vi "Logging Writing Cache.vi"(4 "error in (no error)":errorcluster, 5 "Variable":T2, 6 "Mode":T3, 7 "LoggingDevRef":T1) -> (0 "error out":errorcluster, 1 "Out":T2[](array[typedef]), 3 "LoggingDevRef":T1)   [LabVIEW 2012, in "femtoRoboLib.lvlib"]
uses:
  femtoRoboLib.lvlib
  Controls/Log Entry - Converted.ctl
  Controls/Logging Cache - Mode.ctl
  Controls/LoggingDevRef.ctl
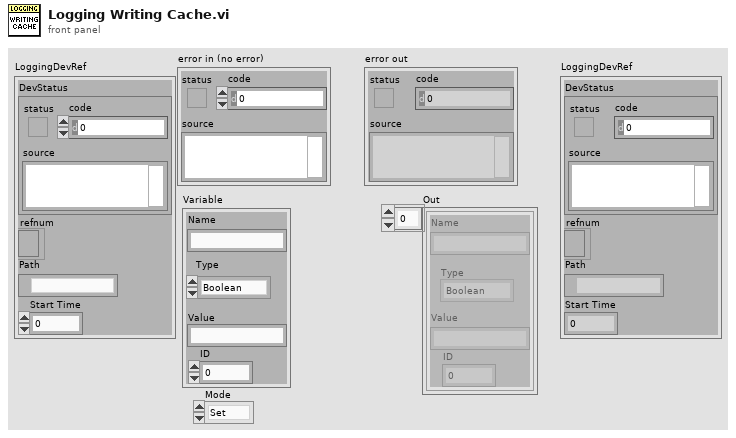
[diagram p1: front panel]
types:
  T1 = typedef "femtoRoboLib.lvlib/LoggingDevRef.ctl" = cluster{"DevStatus":errorcluster, "refnum":refnum<file>, "Path":path, "Start Time":u32}
  T2 = typedef "femtoRoboLib.lvlib/Log Entry - Converted.ctl" = cluster{"Name":string, "Type":enum16{"Boolean", "Numeric", "String", "Boolean Array", "Numeric Array", "String Array"}, "Value":string, "ID":u32}
  T3 = typedef "Logging Cache - Mode.ctl" = enum16{"Set", "Get All", "Get Unsaved", "Get Unsaved and Clear", "Get New", "Get New and Clear"}
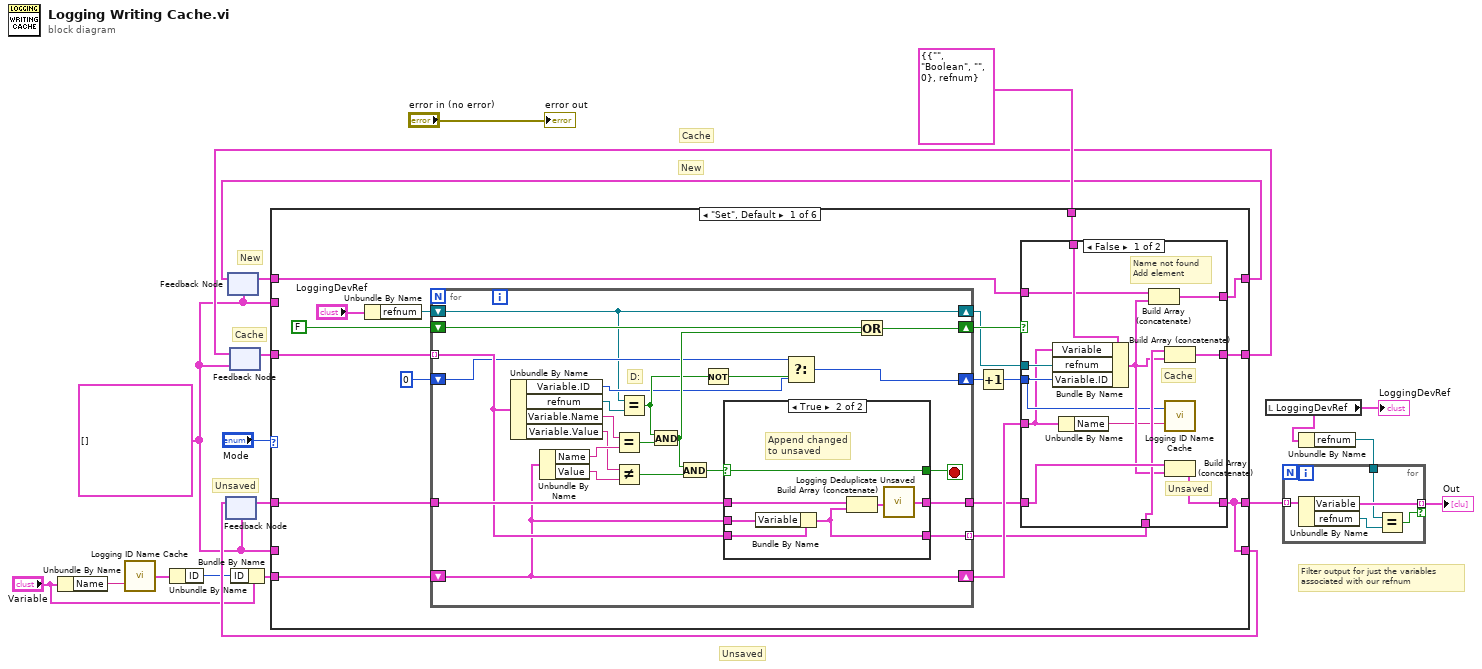
[diagram p0: block diagram]
diagram:
  w7 = cluster{"Variable":T2, "refnum":refnum<file>}[] [] ("Cache")
  # "New"
  # "Cache"
  # "Unsaved"
  # "New"
  # "Cache"
  # "Filter output for just the variables\nassociated with our refnum"
  # "Unsaved"
  n1 = Unbundle By Name("Variable") -> ("Name"=w5:string)
  n2 = call "Logging ID Name Cache.vi"("Name"=w5) -> ("ID/Name"=w4:cluster{"ID":u32, "Name":string})  [unwired: 1 in]
  n3 = Unbundle By Name(w4) -> ("ID"=w2:u32)
  n4 = feedback #1(w7) -> (w18:cluster{"Variable":T2, "refnum":refnum<file>}[])
  n5 = feedback #2(w7) -> (w8:cluster{"Variable":T2, "refnum":refnum<file>}[])
  n6 = feedback #3(w7) -> (w19:cluster{"Variable":T2, "refnum":refnum<file>}[])
  n7 = Bundle By Name(cluster="Variable", "ID"=w2) -> (w1:T2)
  n8 = case shown="\"Set\", Default" "Mode" {
    tunnel: w19 -> [w31 w88 w91 w94 w98 w102]
    tunnel: w18 -> [w38 w89 w92 w95 w99 w103]
    tunnel: [w33 w88 w92 w95 w97 w101] -> w13
    tunnel: w7 -> [_ _ _ w96 _ _]
    tunnel: [w33 w89 w92 w96 w99 w103] -> w16
    tunnel: cluster{"Variable":T2, "refnum":refnum<file>} {"Variable"={"Name"="", "Type"=enum."Boolean", "Value"="", "ID"=0}, "refnum"=refnum} ("Cache Entry") -> [w32 _ _ _ _ _]
    tunnel: [w30 w88 w91 w94 w98 w102] -> w14
    tunnel: w8 -> [w24 w87 w90 w93 w97 w101]
    tunnel: [w25 w87 w90 w93 w97 w100] -> w6
    tunnel: w7 -> [_ _ _ _ _ w100]
    tunnel: w1 -> [w23 _ _ _ _ _]
    frame "Set", Default {
      n9 = Unbundle By Name("LoggingDevRef") -> ("refnum"=w22:refnum<file>)
      n10 = for {
        tunnel: w31 -> [w63] mode=indexing
        tunnel: [w71] -> w34
        tunnel: w38 -> [w72]
        shift-right: [w69] -> w35
        shift-left: FALSE -> [w70]
        tunnel: [w62] -> w29 mode=indexing
        shift-right: [w59] -> w27
        shift-left: u32 0 -> [w56]
        shift-right: [w55] -> w36
        shift-left: w23 -> [w55]
        shift-right: [w54] -> w21
        shift-left: w22 -> [w54]
        stop <- w61 stop-if-true
        # "D:"
        n11 = Unbundle By Name(w63) -> ("Variable.ID"=w57:u32, "refnum"=w68:refnum<file>, "Variable.Name"=w76:string, "Variable.Value"=w74:string)
        n12 = Unbundle By Name(w55) -> ("Name"=w75:string, "Value"=w73:string)
        n13 = Equal?(x=w76, y=w75) -> (x = y?=w67:bool)
        n14 = Not Equal?(x=w74, y=w73) -> (x != y?=w64:bool)
        n15 = Equal?(x=w54, y=w68) -> (x = y?=w60:bool)
        n16 = And(x=w60, y=w67) -> (x .and. y?=w65:bool)
        n17 = And(x=w65, y=w64) -> (x .and. y?=w66:bool)
        n18 = Not(x=w60) -> (.not. x?=w58:bool)
        n19 = case shown="True" w66 {
          selector: w66 -> [w77 w82]
          tunnel: w55 -> [_ w85]
          tunnel: [w79 w80] -> w71
          tunnel: w72 -> [w79 w86]
          tunnel: w63 -> [w78 w84]
          tunnel: [w78 w83] -> w62
          tunnel: [w77 w82] -> w61
          frame False {
          }
          frame True {
            # "Append changed\nto unsaved"
            n20 = Bundle By Name(cluster=w84, "Variable"=w85) -> (w83:cluster{"Variable":T2, "refnum":refnum<file>})
            n21 = Build Array (concatenate)(w86, w83) -> (w81:cluster{"Variable":T2, "refnum":refnum<file>}[])
            n22 = call "Logging Deduplicate Unsaved.vi"("Input"=w81) -> ("Output"=w80:cluster{"Variable":T2, "refnum":refnum<file>}[])
          }
        }
        n23 = Select(t=w56, s=w58, f=w57) -> (s? t:f=w59:u32)
        n24 = Or(x=w70, y=w65) -> (x .or. y?=w69:bool)
      }
      n25 = Increment(x=w27) -> (x+1=w26:u32)
      n26 = case shown="False" w35 {
        tunnel: w36 -> [w40 _]
        tunnel: w34 -> [w50 w53]
        tunnel: [w49 w53] -> w33
        tunnel: w21 -> [w47 _]
        tunnel: w32 -> [w48 _]
        tunnel: [w46 w52] -> w30
        tunnel: w29 -> [w45 w52]
        tunnel: w26 -> [w41 _]
        tunnel: [w44 w51] -> w25
        tunnel: w24 -> [w43 w51]
        frame False {
          # "Cache"
          # "Unsaved"
          # "Name not found\nAdd element"
          n27 = Bundle By Name(cluster=w48, "Variable"=w40, "refnum"=w47, "Variable.ID"=w41) -> (w42:cluster{"Variable":T2, "refnum":refnum<file>})
          n28 = Unbundle By Name(w40) -> ("Name"=w39:string)
          n29 = Build Array (concatenate)(w43, w42) -> (w44:cluster{"Variable":T2, "refnum":refnum<file>}[])
          n30 = Build Array (concatenate)(w45, w42) -> (w46:cluster{"Variable":T2, "refnum":refnum<file>}[])
          n31 = call "Logging ID Name Cache.vi"("Name"=w39, "ID"=w41) -> ()  [unwired: 1 out]
          n32 = Build Array (concatenate)(w50, w42) -> (w49:cluster{"Variable":T2, "refnum":refnum<file>}[])
        }
        frame True {
          # "New"
          # "Cache"
          # "Unsaved"
        }
      }
    }
    frame "Get All" {
      # "New = New"
      # "Unsaved = Unsaved"
      # "Cache = Cache"
      # "Output = Cache"
    }
    frame "Get Unsaved" {
      # "New = New"
      # "Cache = Cache"
      # "Unsaved = Unsaved"
      # "Output = Unsaved"
    }
    frame "Get Unsaved and Clear" {
      # "New = New"
      # "Cache = Cache"
      # "Output = Unsaved"
      # "Unsaved = Empty"
    }
    frame "Get New" {
    }
    frame "Get New and Clear" {
      # "Unsaved = Unsaved"
      # "Output = New"
      # "New = Empty"
      # "Cache = Cache"
    }
  }
  n33 = feedback-in #1(w16) -> ()
  n34 = feedback-in #2(w6) -> ()
  n35 = feedback-in #3(w14) -> ()
  n36 = local read "LoggingDevRef"() -> (w10:T1)
  "LoggingDevRef" <- w10
  n37 = Unbundle By Name(w10) -> ("refnum"=w11:refnum<file>)
  n38 = for {
    tunnel: w13 -> [w108] mode=indexing
    tunnel: [w107] -> w12 mode=indexing if=w106
    tunnel: w11 -> [w105]
    n39 = Unbundle By Name(w108) -> ("Variable"=w107:T2, "refnum"=w104:refnum<file>)
    n40 = Equal?(x=w105, y=w104) -> (x = y?=w106:bool)
  }
  "Out" <- w12
  "error out" <- "error in (no error)"
